vi "Tester.vi"() -> ()   [LabVIEW 2013]
uses:
  <vilib>/vision/NI_Vision_Development_Module.lvlib
panel:
  out "Height Map":T1(plugin-control)
  in  "Grayscale?":bool
  in  "Kernel Size":i32
  out "Image":T1(plugin-control)
  out "error out":errorcluster
  in  "error in (no error)":errorcluster
  in  "Path":path
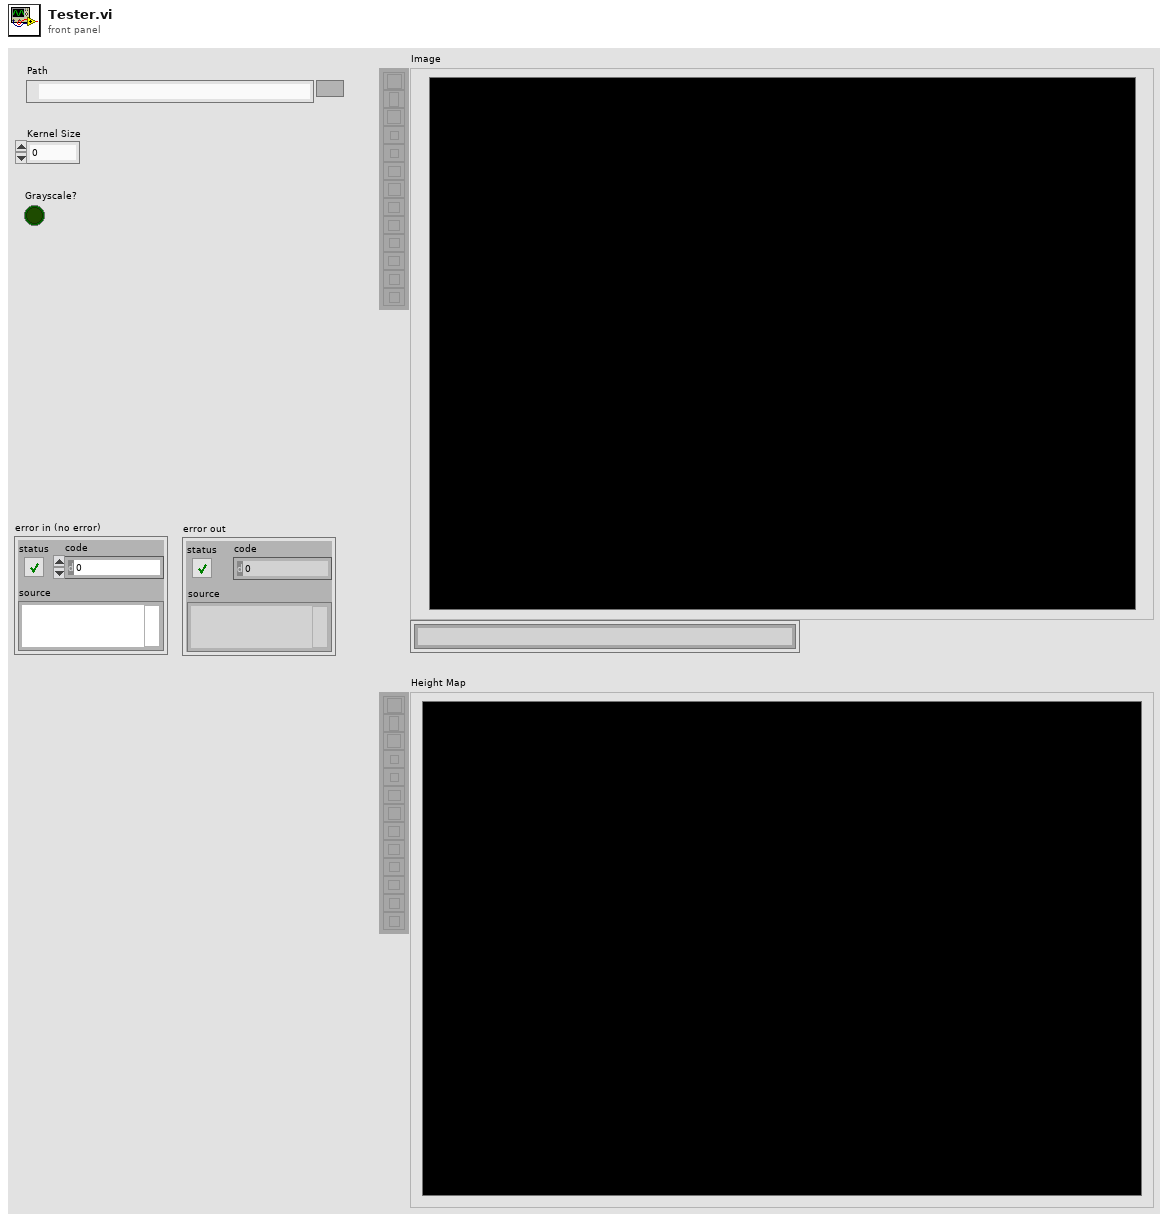
[diagram p1: front panel]
types:
  T1 = typedef "IMAQ Image.ctl" = refnum<image>
  T2 = typedef "Image Type" = u32
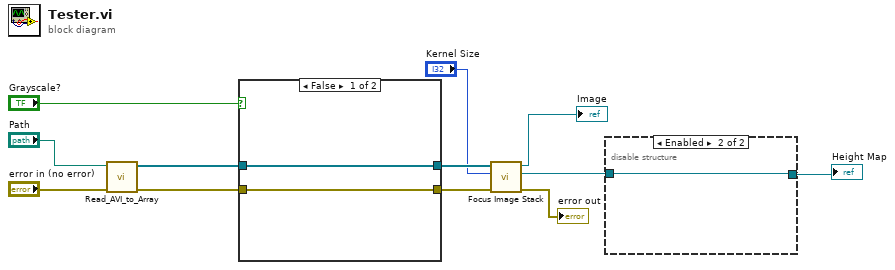
[diagram p0: block diagram]
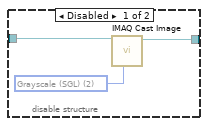
[diagram p2: hidden frame]
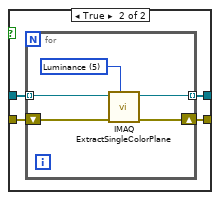
[diagram p3: hidden frame]
diagram:
  n1 = call "Read_AVI_to_Array.vi"("Error in (no error)"="error in (no error)", "AVI Path"="Path") -> ("Error out"=w8:errorcluster, "Image Array"=w1:T1[])  [unwired: 7 in, 1 out]
  n2 = case shown="False" "Grayscale?" {
    tunnel: w8 -> [w13 w18]
    tunnel: w1 -> [w14 w17]
    tunnel: [w14 w16] -> w7
    tunnel: [w13 w15] -> w6
    frame False {
    }
    frame True {
      n3 = for {
        shift-right: [w21] -> w15
        shift-left: w18 -> [w23]
        tunnel: w17 -> [w22] mode=indexing
        tunnel: [w20] -> w16 mode=indexing
        w19 = 5 items=["Red", "Green", "Blue", "Hue", "Saturation", "Luminance", "Value", "Intensity"] ("Color Plane")
        n4 = call "IMAQ ExtractSingleColorPlane"("Color Plane"=w19, "error in (no error)"=w23, "Image Src"=w22) -> ("error out"=w21:errorcluster, "Image Dst Out"=w20:T1)  [unwired: 7 in]
      }
    }
  }
  n5 = call "Focus Image Stack.vi"("error in (no error)"=w6, "Kernel Size"="Kernel Size", "Image Stack"=w7) -> ("error out"=→"error out":errorcluster, "Height Map"=w3:T1, "Focused Image"=→"Image":T1)  [unwired: 6 in]
  n6 = disable-structure shown="Enabled" {
    disable-tunnel: w3 -> [w26 w27]
    disable-tunnel: [w25 w27] -> w2
    frame Disabled {
      w24 = T2 2 items=["Grayscale (U8)", "Grayscale (I16)", "Grayscale (SGL)", "Complex (CSG)", "RGB (U32)", "HSL (U32)", "RGB (U64)", "Grayscale (U16)"] ("Image Type")
      n7 = call "IMAQ Cast Image"("Image Type"=w24, "Image Src"=w26) -> ("Image Dst Out"=w25:T1)  [unwired: 4 in, 5 out]
    }
    frame Enabled {
    }
  }
  "Height Map" <- w2
